vi "read feature list.vi"(11 "Stn# in":string="Stn 1") -> (0 "error out":errorcluster, 1 "Feature list":string[](array[string]), 2 "Stn# out":string, 3 "Refnum out":T1, 5 "table":string[][](array[string]))   [LabVIEW 2015]
uses:
  <vilib>/Utility/config.llb/Config Data RefNum.ctl
  <vilib>/Utility/config.llb/NI_LVConfig.lvlib
panel:
  in  "error in":errorcluster
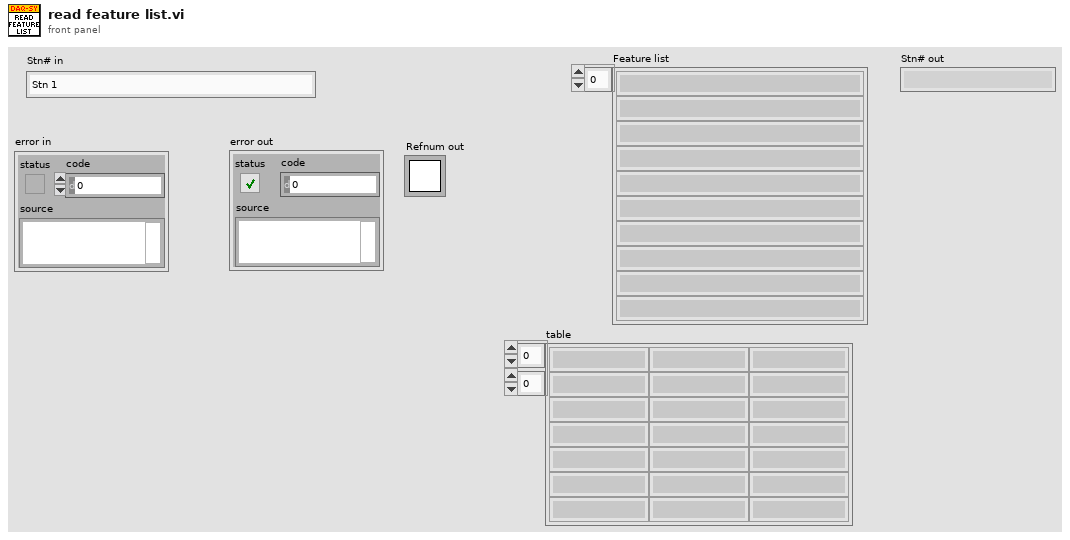
[diagram p1: front panel]
types:
  T1 = typedef "NI_LVConfig.lvlib/Config Data RefNum.ctl" = refnum<k1>
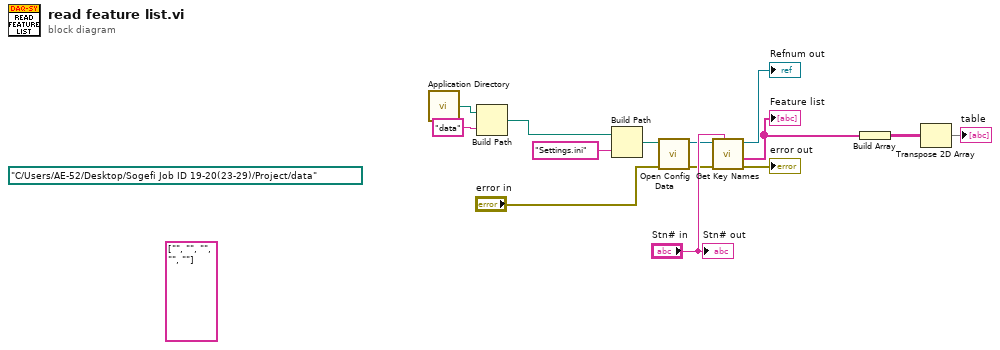
[diagram p0: block diagram]
diagram:
  (unwired) string[] ["", "", "", "", ""]
  (unwired) path "C:/Users/AE-52/Desktop/Sogefi Job ID 19-20(23-29)/Project/data" ("base path")
  n1 = call <vilib>:"Application Directory.vi"() -> ("Application Directory"=w2:path)
  n2 = Build Path(base path=w2, name or relative path="data") -> (appended path=w1:path)
  n3 = Build Path(base path=w1, name or relative path="Settings.ini") -> (appended path=w5:path)
  n4 = call <vilib>:"Open Config Data.vi"("error in (no error)"="error in", "configuration file path"=w5) -> ("error out"=w11:errorcluster, "refnum"=w4:T1)  [unwired: 7 in, 1 out]
  n5 = call <vilib>:"Get Key Names.vi"("section"="Stn# in", "error in (no error)"=w11, "refnum"=w4) -> ("error out"=→"error out":errorcluster, "key names"=w7:string[], "refnum out"=→"Refnum out":T1)  [unwired: 5 in, 1 out]
  "Feature list" <- w7
  n6 = Build Array(w7) -> (w8:string[][])
  n7 = Transpose 2D Array(2D array=w8) -> (transposed array=→"table":string[][])
  "Stn# out" <- "Stn# in"
